vi "InitMainSize.vi"(1 "VI Refnum In":refnum<vi>) -> (0 "VI Refnum Out":refnum<vi>)   [LabVIEW 2010]
panel:
  out "Array 3":u32[](array[numeric])
  out "Array 2":string[](array[string])
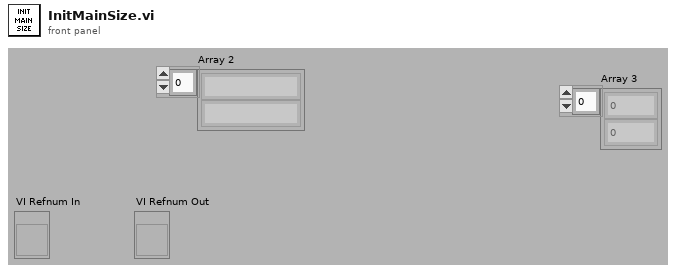
[diagram p1: front panel]
types:
  T1 = typedef "LVRectTypeDef.ctl" = cluster{"left":i16, "top":i16, "right":i16, "bottom":i16}
  T2 = typedef "LVBoundsTypeDef.ctl" = cluster{"Width":u32, "Height":u32}
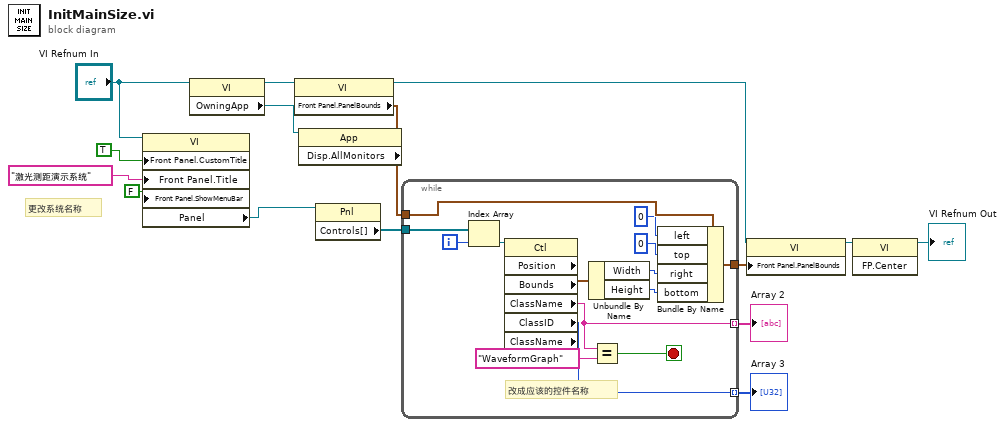
[diagram p0: block diagram]
diagram:
  # "更改系统名称"
  n1 = property class="VI"(reference="VI Refnum In", "Front Panel.CustomTitle"=TRUE ("Front Panel Window:Custom Title"), "Front Panel.Title"="激光测距演示系统" ("Front Panel Window:Title"), "Front Panel.ShowMenuBar"=FALSE ("Front Panel Window:Show Menu Bar")) -> ("Panel"=w10:refnum<vi>)  [unwired: 1 in, 2 out]
  n2 = property class="VI"(reference="VI Refnum In") -> (reference out=w15:refnum<vi>, "OwningApp"=w14:refnum<vi>)  [unwired: 1 in, 1 out]
  n3 = property class="VI"(reference=w15) -> (reference out=w5:refnum<vi>, "Front Panel.PanelBounds"=w6:T1)  [unwired: 1 in, 1 out]
  n4 = property class="App" props=["Disp.AllMonitors"](reference=w14) -> ()  [unwired: 1 in, 3 out]
  n5 = property class="Pnl"(reference=w10) -> ("Controls[]"=w9:refnum<vi>[])  [unwired: 1 in, 2 out]
  n6 = while {
    tunnel: w9 -> [w24]
    tunnel: [w27] -> w7 mode=indexing
    tunnel: w6 -> [w29]
    tunnel: [w28] -> w1
    tunnel: [w21] -> w4 mode=indexing
    i -> [w23]
    stop <- w25 stop-if-true
    # "改成应该的控件名称"
    n7 = Index Array(array=w24, index=w23) -> (element=w22:refnum<vi>)
    n8 = property class="Ctl" props=["Position", "Bounds", "ClassName", "ClassID", "ClassName"](reference=w22) -> ("Bounds"=w20:T2, "ClassName"=w27:string, "ClassID"=w21:u32)  [unwired: 1 in, 4 out]
    n9 = Unbundle By Name(w20) -> ("Width"=w17:u32, "Height"=w16:u32)
    n10 = Equal?(x=w27, y="WaveformGraph") -> (x = y?=w25:bool)
    n11 = Bundle By Name(cluster=w29, "left"=i16 0, "top"=i16 0, "right"=w17, "bottom"=w16) -> (w28:T1)
  }
  "Array 2" <- w7
  "Array 3" <- w4
  n12 = property class="VI"(reference=w5, "Front Panel.PanelBounds"=w1) -> (reference out=w3:refnum<vi>)  [unwired: 1 in, 1 out]
  n13 = invoke class="VI" method="FP.Center"(reference=w3) -> (reference out=→"VI Refnum Out":refnum<vi>)  [unwired: 2 in, 2 out]
